vi "Set_VI_Ref.vi"(8 "error in (no error)":errorcluster, 11 "Class 3 in":refnum<class "Class 3.lvclass">) -> (0 "error out":errorcluster, 2 "Core_Reference_VI out":refnum<vi>, 3 "Class 3 out":refnum<class "Class 3.lvclass">)   [LabVIEW 2021, in "Class 3.lvclass"]
uses:
  Class 3.lvclass
  Modules/Sample_Panel_3.vi
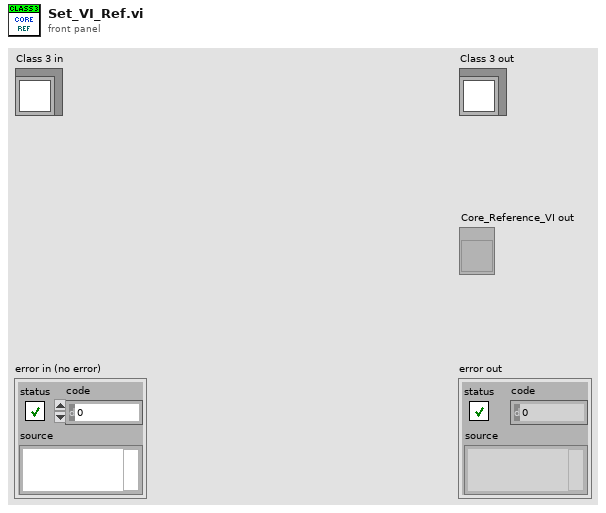
[diagram p1: front panel]
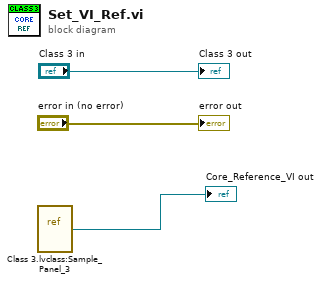
[diagram p0: block diagram]
diagram:
  n1 = vi-ref "Class 3.lvclass:Sample_Panel_3.vi"() -> (→"Core_Reference_VI out":refnum<vi>)
  "error out" <- "error in (no error)"
  "Class 3 out" <- "Class 3 in"
